vi "lxw parse range.vi"(0 "range_str":string, 1 "last_col":u16, 5 "first_row":u32, 7 "first_col":u16, 9 "last_row":u32, 11 "error in (no error)":errorcluster) -> (3 "last_col out":u16, 6 "first_row out":u32, 8 "first_col out":u16, 10 "last_row out":u32, 15 "error out":errorcluster)   [LabVIEW 2015, in "xlsxwriter.lvlib"]
doc: "void lxw_parse_range(const char *range_str, lxw_row_t *first_row, lxw_col_t *first_col, lxw_row_t *last_row, lxw_col_t *last_col);"
uses:
  xlsxwriter.lvlib
  xlsxwriter.dll
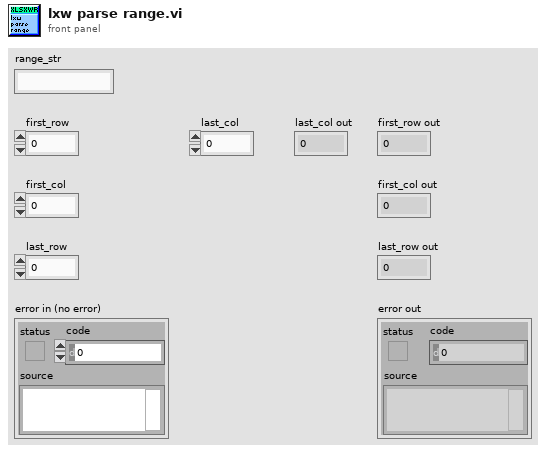
[diagram p1: front panel]
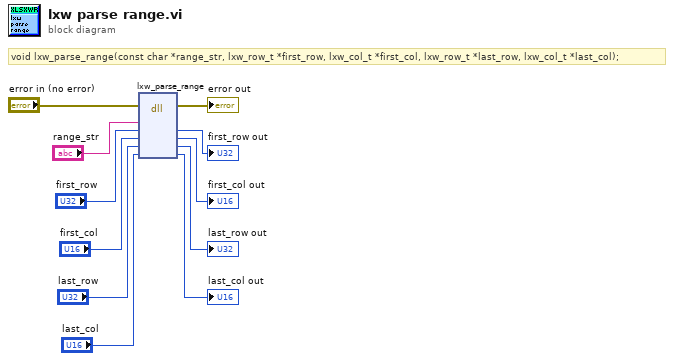
[diagram p0: block diagram]
diagram:
  # "void lxw_parse_range(const char *range_str, lxw_row_t *first_row, lxw_col_t *first_col, lxw_row_t *last_row, lxw_col_t *last_col);"
  n1 = dll-call lib="C:/Users/WDAGUtilityAccount/Desktop/lv_vis_added_cell/xlsxwriter.*" fn="lxw_parse_range"(error in="error in (no error)", "range_str"="range_str", "first_row"="first_row", "first_col"="first_col", "last_row"="last_row", "last_col"="last_col") -> (error out=→"error out":errorcluster, "first_row"=→"first_row out":u32, "first_col"=→"first_col out":u16, "last_row"=→"last_row out":u32, "last_col"=→"last_col out":u16)  [unwired: 4 in, 1 out]
